vi "rotm_obs_new.vi"(6 "angle[rad]":dbl, 7 "reverse":bool, 8 "y0":dbl, 9 "x0":dbl, 10 "y":dbl[](array[numeric]), 11 "x":dbl[](array[numeric])) -> (0 "rot*[x-x0;y-y0]":dbl[][](array[numeric]), 2 "rot*(y-y0) 2":dbl[](array[numeric]), 3 "rot*(x-x0)":dbl[](array[numeric]), 5 "rot*(y-y0)":dbl[](array[numeric]))   [LabVIEW 2015]
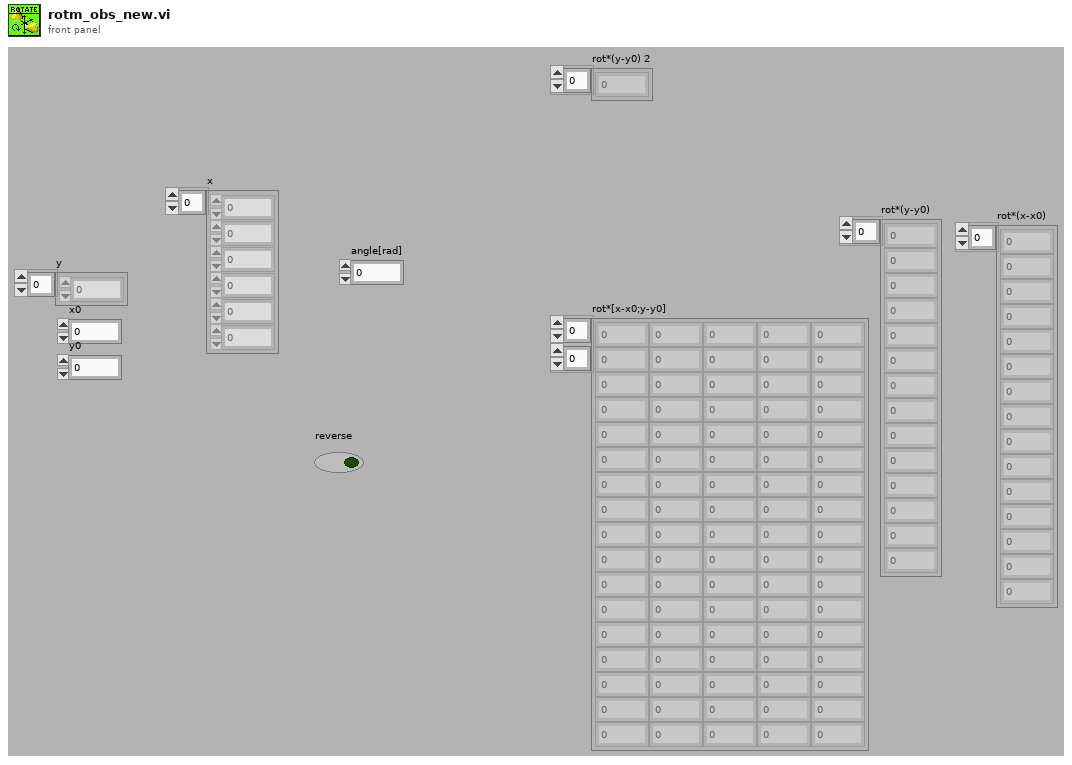
[diagram p1: front panel]
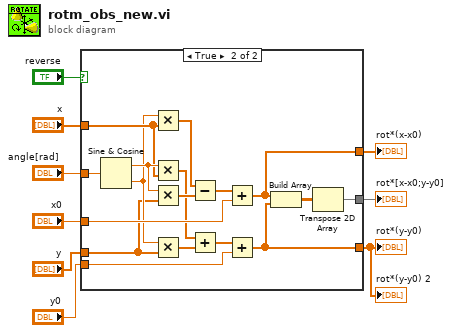
[diagram p0: block diagram]
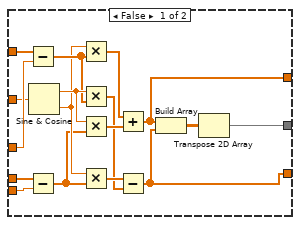
[diagram p2: hidden frame]
diagram:
  n1 = case shown="True" "reverse" {
    tunnel: "angle[rad]" -> [w22 w43]
    tunnel: "x" -> [w26 w37]
    tunnel: "x0" -> [w25 w39]
    tunnel: "y0" -> [w23 w31]
    tunnel: "y" -> [w24 w35]
    tunnel: [w10 w27] -> w4
    tunnel: [w13 w30] -> w3
    tunnel: [w12 w29] -> w1
    frame False {
      n2 = Subtract(x=w26, y=w25) -> (x-y=w18:dbl[])
      n3 = Subtract(x=w24, y=w23) -> (x-y=w16:dbl[])
      n4 = Sine & Cosine(0:w22) -> (1:w19:dbl, 2:w17:dbl)
      n5 = Multiply(x=w17, y=w18) -> (x*y=w21:dbl[])
      n6 = Multiply(x=w19, y=w18) -> (x*y=w14:dbl[])
      n7 = Multiply(x=w19, y=w16) -> (x*y=w20:dbl[])
      n8 = Multiply(x=w17, y=w16) -> (x*y=w15:dbl[])
      n9 = Add(x=w21, y=w20) -> (x+y=w13:dbl[])
      n10 = Subtract(x=w15, y=w14) -> (x-y=w12:dbl[])
      n11 = Build Array(w13, w12) -> (w11:dbl[][])
      n12 = Transpose 2D Array(2D array=w11) -> (transposed array=w10:dbl[][])
    }
    frame True {
      n13 = Sine & Cosine(0:w43) -> (1:w38:dbl, 2:w36:dbl)
      n14 = Multiply(x=w36, y=w37) -> (x*y=w42:dbl[])
      n15 = Multiply(x=w38, y=w37) -> (x*y=w34:dbl[])
      n16 = Multiply(x=w38, y=w35) -> (x*y=w41:dbl[])
      n17 = Multiply(x=w36, y=w35) -> (x*y=w33:dbl[])
      n18 = Subtract(x=w42, y=w41) -> (x-y=w40:dbl[])
      n19 = Add(x=w34, y=w33) -> (x+y=w32:dbl[])
      n20 = Add(x=w40, y=w39) -> (x+y=w30:dbl[])
      n21 = Add(x=w32, y=w31) -> (x+y=w29:dbl[])
      n22 = Build Array(w30, w29) -> (w28:dbl[][])
      n23 = Transpose 2D Array(2D array=w28) -> (transposed array=w27:dbl[][])
    }
  }
  "rot*[x-x0;y-y0]" <- w4
  "rot*(x-x0)" <- w3
  "rot*(y-y0)" <- w1
  "rot*(y-y0) 2" <- w1
